vi "DDS_server.vi"() -> ()   [LabVIEW 2014, in "Experiment.lvclass"]
uses:
  Experiment.lvclass
  TCP_IP/TCP_IP.lvclass
  Globals.vi
  <vilib>/platform/TimedLoop/XDataNode/XDataNode.xnode
  <vilib>/Platform/TimedLoop/XDataNode/nitl_modes.ctl
  <vilib>/Platform/TimedLoop/XDataNode/XDNodeRunTimeDep.lvlib
  <vilib>/Platform/TimedLoop/XDataNode/wakeup.ctl
  <vilib>/Platform/TimedLoop/XDataNode/timing_clust.ctl
  DDS/DDS.lvclass
  <vilib>/ni845x/ni845x.llb/ni845xControl.ctl
  DDS/DDS Library/Controls/DDS Box Device Reference.ctl
  DDS/DDS Library/DDS.lvlib
  DDS/DDS Library/Controls/DDS Channel Parameters.ctl
  DDS/DDS Library/Controls/DDS RAM Destination.ctl
  DDS/DDS Library/Controls/DDS RAM Mode.ctl
  DDS/DDS Library/Controls/DDS RAM Timestep.ctl
  DDS/DDS Library/Controls/DDS Profile.ctl
  DDS/DDS Library/Controls/DDS Profile Array.ctl
  DDS/DDS Library/Controls/DDS Channel.ctl
  DDS/DDS Library/Controls/DDS Channel Array.ctl
  DDS/DDS Library/Controls/DDS Box Cluster.ctl
  DDS/DDS Library/Controls/DDS Box Array.ctl
  DDS/DDS_Settings_Cluster.ctl
panel:
  in  "IP address to listen on\n(blank for all networks)":string
  out "DDS Settings":T1={"Enable DDS"=TRUE, "Array of DDS Boxes"=[{"DDS box device reference"={"NI USB-8451 device reference"="USB0::0x3923::0x7166::01574F57::RAW", "DIO port"=0, "Serial Clock Rate [kHz]"=1000}, "Array of DDS Channels (4)"=[{"Power"=FALSE, "Channel Parameters"={"Ref Clock Rate [MHz]"=1000.0, "Full Scale Output\nPower [dBm]"=0.0}, "RAM Enable"=FALSE, "RAM Dest Type"=enum."Frequency", "RAM Default"={"Frequency [MHz]"=0.0, "Amplitude [dBm]"=0.0, "Phase Offset [rad]"=0.0}, "Array of DDS Profiles (8)"=[], "Description"=""}, {"Power"=FALSE, "Channel Parameters"={"Ref Clock Rate [MHz]"=1000.0, "Full Scale Output\nPower [dBm]"=0.0}, "RAM Enable"=FALSE, "RAM Dest Type"=enum."Frequency", "RAM Default"={"Frequency [MHz]"=0.0, "Amplitude [dBm]"=0.0, "Phase Offset [rad]"=0.0}, "Array of DDS Profiles (8)"=[], "Description"=""}, {"Power"=FALSE, "Channel Parameters"={"Ref Clock Rate [MHz]"=1000.0, "Full Scale Output\nPower [dBm]"=0.0}, "RAM Enable"=FALSE, "RAM Dest Type"=enum."Frequency", "RAM Default"={"Frequency [MHz]"=0.0, "Amplitude [dBm]"=0.0, "Phase Offset [rad]"=0.0}, "Array of DDS Profiles (8)"=[], "Description"=""}, {"Power"=FALSE, "Channel Parameters"={"Ref Clock Rate [MHz]"=1000.0, "Full Scale Output\nPower [dBm]"=0.0}, "RAM Enable"=FALSE, "RAM Dest Type"=enum."Frequency", "RAM Default"={"Frequency [MHz]"=0.0, "Amplitude [dBm]"=0.0, "Phase Offset [rad]"=0.0}, "Array of DDS Profiles (8)"=[], "Description"=""}], "Enable"=TRUE, "Description"=""}, {"DDS box device reference"={"NI USB-8451 device reference"="USB0::0x3923::0x7166::01574FA5::RAW", "DIO port"=0, "Serial Clock Rate [kHz]"=1000}, "Array of DDS Channels (4)"=[{"Power"=FALSE, "Channel Parameters"={"Ref Clock Rate [MHz]"=1000.0, "Full Scale Output\nPower [dBm]"=0.0}, "RAM Enable"=FALSE, "RAM Dest Type"=enum."Frequency", "RAM Default"={"Frequency [MHz]"=0.0, "Amplitude [dBm]"=0.0, "Phase Offset [rad]"=0.0}, "Array of DDS Profiles (8)"=[], "Description"=""}, {"Power"=FALSE, "Channel Parameters"={"Ref Clock Rate [MHz]"=1000.0, "Full Scale Output\nPower [dBm]"=0.0}, "RAM Enable"=FALSE, "RAM Dest Type"=enum."Frequency", "RAM Default"={"Frequency [MHz]"=0.0, "Amplitude [dBm]"=0.0, "Phase Offset [rad]"=0.0}, "Array of DDS Profiles (8)"=[], "Description"=""}, {"Power"=FALSE, "Channel Parameters"={"Ref Clock Rate [MHz]"=1000.0, "Full Scale Output\nPower [dBm]"=0.0}, "RAM Enable"=FALSE, "RAM Dest Type"=enum."Frequency", "RAM Default"={"Frequency [MHz]"=0.0, "Amplitude [dBm]"=0.0, "Phase Offset [rad]"=0.0}, "Array of DDS Profiles (8)"=[], "Description"=""}, {"Power"=FALSE, "Channel Parameters"={"Ref Clock Rate [MHz]"=1000.0, "Full Scale Output\nPower [dBm]"=0.0}, "RAM Enable"=FALSE, "RAM Dest Type"=enum."Frequency", "RAM Default"={"Frequency [MHz]"=0.0, "Amplitude [dBm]"=0.0, "Phase Offset [rad]"=0.0}, "Array of DDS Profiles (8)"=[], "Description"=""}], "Enable"=TRUE, "Description"=""}]} {"Array of DDS Boxes"."Array of DDS Channels (4)"."Channel Parameters"."Ref Clock Rate [MHz]" min=0.0}
  in  "port":u16=9001
  out "Log History":string
  in  "Clear Log":bool
  out "Done":bool
  in  "Restart":bool
  out "Log":string
  in  "Stop":bool
  # "f/f/A"
  # "Mag"
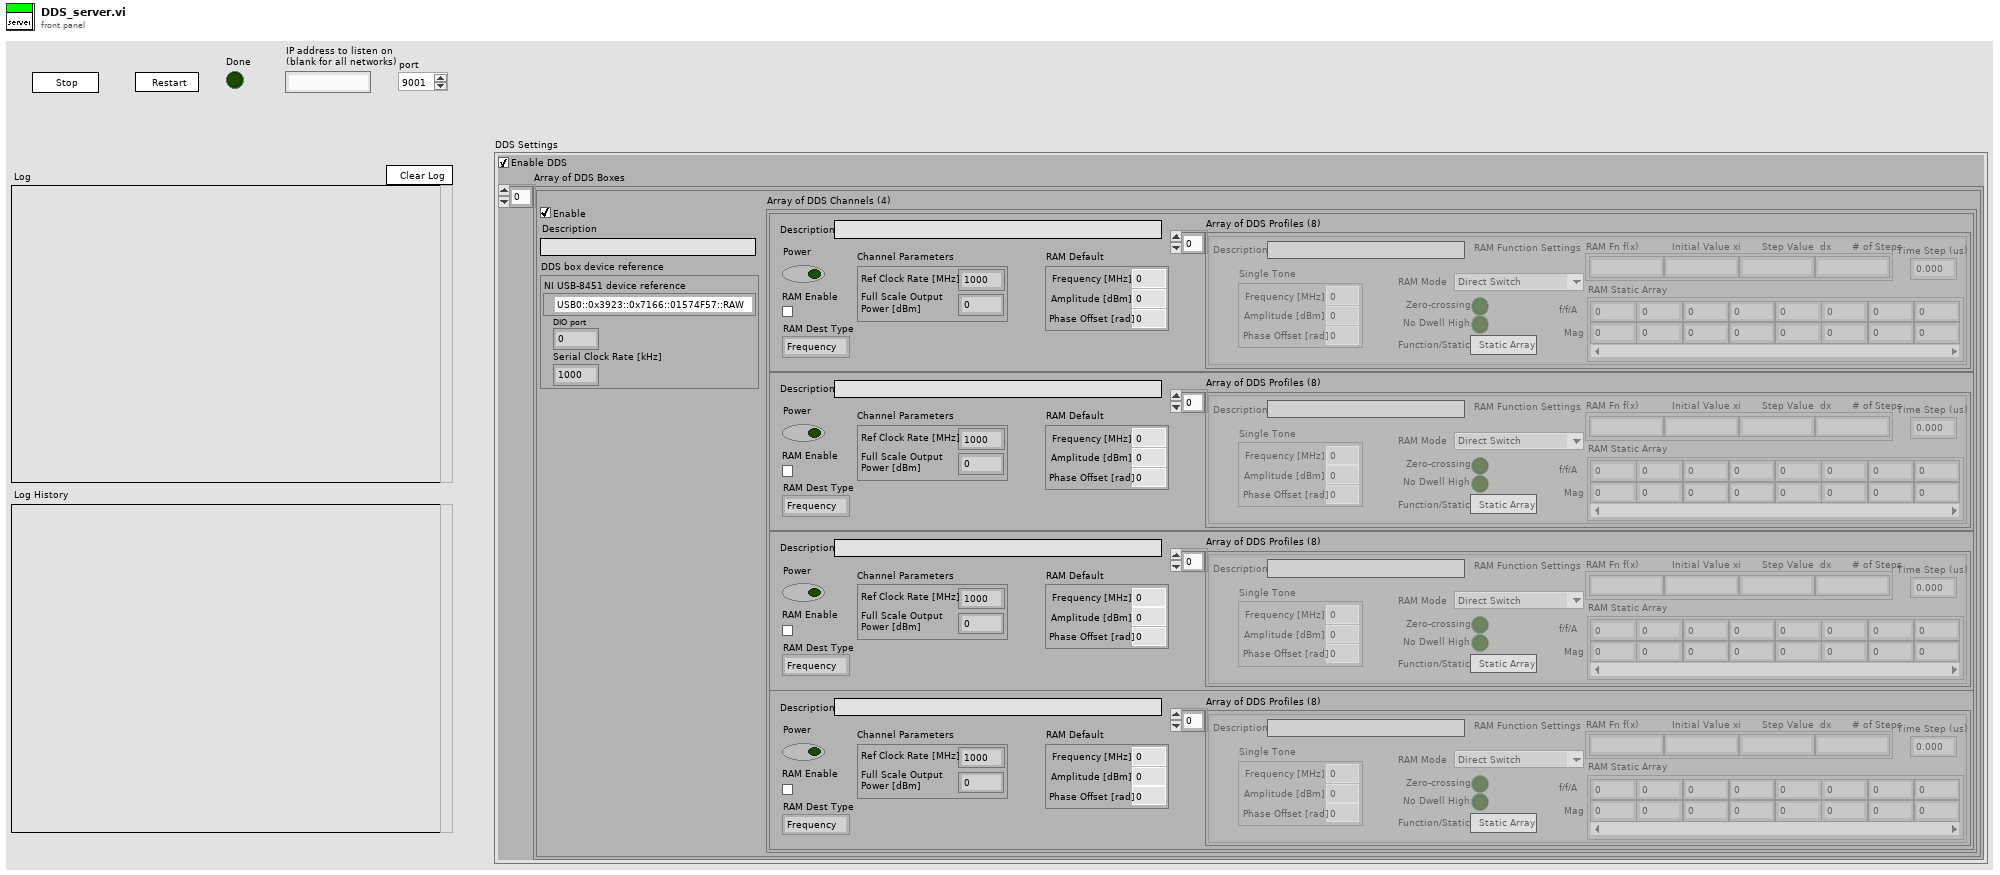
[diagram p1: front panel]
types:
  T1 = typedef "DDS.lvclass/DDS_Settings_Cluster.ctl" = cluster{"Enable DDS":bool, "Array of DDS Boxes":T2}
  T2 = typedef "DDS.lvlib/DDS Box Array.ctl" = T3[]
  T3 = typedef "DDS.lvlib/DDS Box Cluster.ctl" = cluster{"DDS box device reference":T4, "Array of DDS Channels (4)":T6, "Enable":bool, "Description":string}
  T4 = typedef "DDS.lvlib/DDS Box Device Reference.ctl" = cluster{"NI USB-8451 device reference":T5, "DIO port":u8, "Serial Clock Rate [kHz]":u16}
  T5 = typedef "ni845xControl.ctl" = refnum<k21>
  T6 = typedef "DDS.lvlib/DDS Channel Array.ctl" = T7[]
  T7 = typedef "DDS.lvlib/DDS Channel.ctl" = cluster{"Power":bool, "Channel Parameters":T8, "RAM Enable":bool, "RAM Dest Type":T9, "RAM Default":cluster{"Frequency [MHz]":dbl, "Amplitude [dBm]":dbl, "Phase Offset [rad]":dbl}, "Array of DDS Profiles (8)":T10, "Description":string}
  T8 = typedef "DDS.lvlib/DDS Channel Parameters.ctl" = cluster{"Ref Clock Rate [MHz]":dbl, "Full Scale Output\nPower [dBm]":dbl}
  T9 = typedef "DDS.lvlib/DDS RAM Destination.ctl" = enum16{"Frequency", "Phase", "Amplitude", "Polar"}
  T10 = typedef "DDS.lvlib/DDS Profile Array.ctl" = T11[]
  T11 = typedef "DDS.lvlib/DDS Profile.ctl" = cluster{"Single Tone":cluster{"Frequency [MHz]":dbl, "Amplitude [dBm]":dbl, "Phase Offset [rad]":dbl}, "RAM Mode ":T12, "Zero-crossing":bool, "No Dwell High":bool, "Function/Static":bool, "RAM Function Settings":string[], "RAM Static Array":dbl[][], "Description":string, "Time Step (us)":T13}
  T12 = typedef "DDS.lvlib/DDS RAM mode.ctl" = enum16{"Direct Switch", "Ramp Up", "Bidirectional Ramp", "Continuous Bidirectional Ramp", "Continuous Recirculate", "Direct Switch 2", "Direct Switch 3", "Direct Switch 4"}
  T13 = typedef "DDS.lvlib/DDS RAM Timestep.ctl" = dbl
  T14 = typedef "XDNodeRunTimeDep.lvlib/timing_clust.ctl" = cluster{"Expected End [f-1]":u64, "Actual End [f-1]":u64, "Finished Late? [f-1]":bool, "Expected End [i-1]":u64, "Actual End [i-1]":u64, "Finished Late? [i-1]":bool, "Expected Start [i]":u64, "Actual Start [i]":u64, "Expected Start [f]":u64, "Actual Start [f]":u64, "Source Name":string, "Structure Name":string, "Period":i64, "Deadline":i64, "Offset":i64, "Start":i64, "Priority":i32, "Timeout":i32, "Mode":T15, "Wakeup Reason":T16, "Error":errorcluster, "Source Type":string, "Secondary Source Type":string, "Global End Time":u64, "Global Start Time":u64, "Frame Duration":u64, "Iteration Duration":u64, "Assigned CPU":i32, "I/O Scan Engine Mode":u32}
  T15 = typedef "XDNodeRunTimeDep.lvlib/nitl_modes.ctl" = enum32{"No Change", "Process missed periods, maintain original phase", "Discard missed periods, maintain original phase", "Process missed periods, ignore original phase", "Discard missed periods, ignore original phase"}
  T16 = typedef "XDNodeRunTimeDep.lvlib/wakeup.ctl" = enum32{"Normal", "Aborted", "Asynchronous wakeup", "Timing source error", "Timed loop error", "Timeout"}
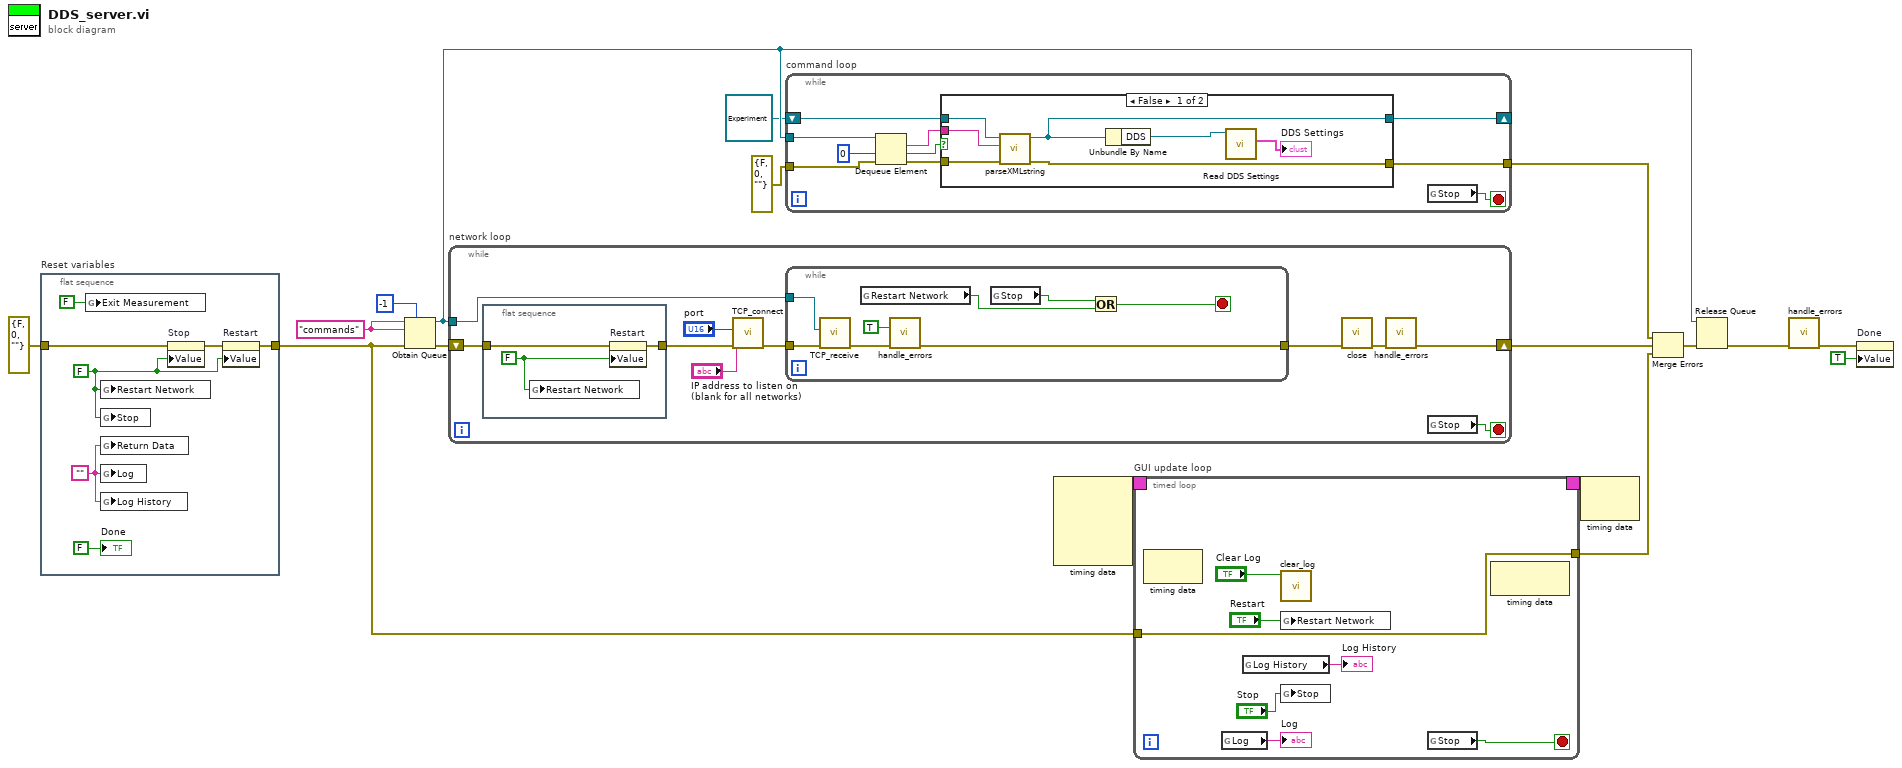
[diagram p0: block diagram]
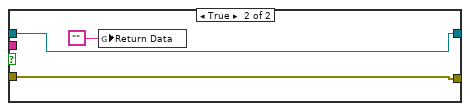
[diagram p2: hidden frame]
diagram:
  w17 = "commands" ("name (unnamed)")
  n1 = flat-sequence "Reset variables" {
    tunnel: [w20] -> w6
    tunnel: errorcluster {"status"=FALSE, "code"=0, "source"=""} ("error in (no error)") -> [w22]
    frame #0 {
      w18 = ""
      w21 = FALSE ("Stop")
      n2 = global write "Globals.vi" "Exit Measurement"(FALSE ("Exit Measurement")) -> ()
      n3 = global write "Globals.vi" "Restart Network"(w21) -> ()
      n4 = global write "Globals.vi" "Stop"(w21) -> ()
      n5 = global write "Globals.vi" "Return Data"(w18) -> ()
      n6 = global write "Globals.vi" "Log"(w18) -> ()
      n7 = global write "Globals.vi" "Log History"(w18) -> ()
      n8 = property on="Stop" class="Bool (strict)"(error in=w22, "Value"=w21) -> (error out=w24:errorcluster)  [unwired: 1 in, 1 out]
      n9 = property on="Restart" class="Bool (strict)"(error in=w24, "Value"=w21) -> (error out=w20:errorcluster)  [unwired: 1 in, 1 out]
      "Done" <- FALSE ("Done")
    }
  }
  n10 = Obtain Queue(max queue size (-1, unlimited)=-1, name (unnamed)=w17, element data type=w17, error in (no error)=w6) -> (queue out=w10:refnum<queue>, error out=w16:errorcluster)  [unwired: 1 in, 1 out]
  n11 = while "network loop" {
    shift-right: [w34] -> w9
    shift-left: w16 -> [w27]
    tunnel: w10 -> [w33]
    stop <- w31 stop-if-true
    n12 = flat-sequence {
      tunnel: [w36] -> w28
      tunnel: w27 -> [w37]
      frame #0 {
        w35 = FALSE ("Restart")
        n13 = global write "Globals.vi" "Restart Network"(w35) -> ()
        n14 = property on="Restart" class="Bool (strict)"(error in=w37, "Value"=w35) -> (error out=w36:errorcluster)  [unwired: 1 in, 1 out]
      }
    }
    n15 = call "TCP_connect.vi"("error in (no error)"=w28, "IP"="IP address to listen on\n(blank for all networks)", "port"="port") -> ("error out"=w29:errorcluster)  [unwired: 8 in]
    n16 = while {
      tunnel: w29 -> [w43]
      tunnel: [w45] -> w32
      tunnel: w33 -> [w44]
      stop <- w42 stop-if-true
      n17 = call "TCP_receive.vi"("error in (no error)"=w43, "queue"=w44) -> ("error out"=w39:errorcluster)  [unwired: 9 in]
      n18 = global read "Globals.vi" "Restart Network"() -> (w40:bool)
      n19 = call "handle_errors.vi"("Restart Network"=TRUE, "error in (no error)"=w39) -> ("error out"=w45:errorcluster)  [unwired: 13 in]
      n20 = global read "Globals.vi" "Stop"() -> (w41:bool)
      n21 = Or(x=w41, y=w40) -> (x .or. y?=w42:bool)
    }
    n22 = call "close.vi"("error in (no error)"=w32) -> ("error out"=w30:errorcluster)  [unwired: 10 in]
    n23 = call "handle_errors.vi"("error in (no error)"=w30) -> ("error out"=w34:errorcluster)  [unwired: 14 in]
    n24 = global read "Globals.vi" "Stop"() -> (w31:bool)
  }
  n25 = while "command loop" {
    tunnel: w10 -> [w55]
    tunnel: errorcluster {"status"=FALSE, "code"=0, "source"=""} ("error constant") -> [w54]
    tunnel: [w46] -> w13
    shift-right: [w48] -> _
    shift-left: refnum<class "Experiment.lvclass"> refnum ("Experiment.lvclass") -> [w49]
    stop <- w47 stop-if-true
    n26 = Dequeue Element(queue=w55, timeout in ms (-1)=0, error in (no error)=w54) -> (element=w51:string, timed out?=w52:bool, error out=w53:errorcluster)  [unwired: 1 out]
    n27 = case shown="False" w52 {
      tunnel: [w62 w65] -> w46
      tunnel: w53 -> [w59 w65]
      tunnel: w51 -> [w61 _]
      tunnel: w49 -> [w60 w64]
      tunnel: [w58 w64] -> w48
      frame False {
        n28 = call "parseXMLstring.vi"("error in (no error)"=w59, "Node Value"=w61, "Experiment.lvclass (in)"=w60) -> ("error out"=w62:errorcluster, "Experiment.lvclass"=w58:refnum<class "Experiment.lvclass">)  [unwired: 7 in]
        n29 = Unbundle By Name(w58) -> ("DDS"=w57:refnum<class "DDS.lvclass">)
        n30 = call-dynamic "Read DDS Settings.vi"("DDS in"=w57) -> ("DDS Settings"=→"DDS Settings":T1)  [unwired: 8 in, 2 out]
      }
      frame True {
        n31 = global write "Globals.vi" "Return Data"("") -> ()
      }
    }
    n32 = global read "Globals.vi" "Stop"() -> (w47:bool)
  }
  n33 = node-c288() -> (w2:T14)  [unwired: 4 in]
  n34 = timed-loop "GUI update loop" {
    tunnel: w6 -> [w68]
    tunnel: [w68] -> w5
    timing: w2 -> [_]
    timing-out: [_] -> w1
    stop <- w69 stop-if-true
    n35 = node-c288() -> ()  [unwired: 1 in, 1 out]
    n36 = global read "Globals.vi" "Log"() -> (→"Log":string)
    n37 = global read "Globals.vi" "Log History"() -> (→"Log History":string)
    n38 = call "clear_log.vi"("clear log?"="Clear Log") -> ()  [unwired: 10 in, 1 out]
    n39 = global write "Globals.vi" "Restart Network"("Restart") -> ()
    n40 = global write "Globals.vi" "Stop"("Stop") -> ()
    n41 = global read "Globals.vi" "Stop"() -> (w69:bool)
    n42 = node-c288() -> ()  [unwired: 1 in, 1 out]
  }
  n43 = node-c288(w1) -> ()  [unwired: 1 out]
  n44 = Merge Errors(w13, w9, w5) -> (w12:errorcluster)
  n45 = Release Queue(queue=w10, error in (no error)=w12) -> (error out=w11:errorcluster)  [unwired: 1 in, 2 out]
  n46 = call "handle_errors.vi"("error in (no error)"=w11) -> ("error out"=w4:errorcluster)  [unwired: 14 in]
  n47 = property on="Done" class="Bool (strict)"(error in=w4, "Value"=TRUE ("Done")) -> ()  [unwired: 1 in, 2 out]
